vi "FUG_PowerSupply.SetCurrent.vi"(0 "i ref in":refnum<vi>, 2 "value":dbl, 5 "error in (no error)":errorcluster, 7 "channel":i32) -> (14 "i ref out":refnum<vi>, 19 "error out (no error)":errorcluster)   [LabVIEW 2014, in "FUG_PowerSupply.lvlib"]
doc: "This VI calculates the right current from the DB values, saves the actual set current to the I-Attribute and set´s the Set Current-Service."
uses:
  FUG_PowerSupply.lvlib
  CS_Core/CSSystem/CoreDefs/CoreDefs.error_type.ctl
  CS_Core/CSSystem/CoreDefs/CoreDefs.error_severity.ctl
  CS_Core/CSApplicationBaseClasses/PSChannelBase/PSChannelBase.directionType.ctl
  CS_Core/CSApplicationBaseClasses/PSChannelBase/PSChannelBase.serviceType.ctl
  CSlibraries/UtilityLib/UtilityLib.valueStatus.ctl
  CS_Core/CSSystem/CoreLib/CoreLib.lvlib
  CSlibraries/UtilityLib/UtilityLib.lvlib
  CS_Core/CSApplicationBaseClasses/PSChannelBase/PSChannelBase.lvlib
  CSlibraries-extern/DimLVEvent/LVDimInterface/LVDimInterface.lvlib
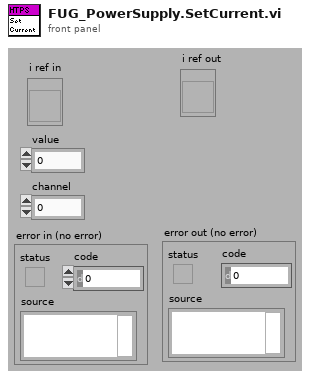
[diagram p1: front panel]
types:
  T1 = typedef "CoreDefs.error_severity.ctl" = enum16{"undefined", "information", "warning", "error", "fatal"}
  T2 = typedef "CoreDefs.error_type.ctl" = enum16{"no error", "can't load process", "can't unload process", "process does not exist", "can't install process", "can't remove process", "unknown function", "time out", "can't execute function", "duplicate queue name", "super not found", "caller queue invalid", "can't ping process", "unknown error", "VISA Error", "VISA timeout", "GPIB timeout", "GPIB error", "communication error", "data type mismatch", "can't read data from OPC server", "can't write data to OPC server", "OET error", "function not implemented", "process already exists", "invalid Shared Variable name", "error writing Shared Variable", "error reading Shared Variable", "invalid client name", "corrupt database", "unknown class", "call not authorized", "parameter out of range", "OET timeout: can't get data to modify", "invalid queue name", "requested operation incompatible with current state", "event undefined", "event disabled", "state undefined", "caller is not a friend", "EventBuilder: bad eventID", "EventBuilder: no DAQ devices", "a thread must not stop itself", "UNUSED ELEMENT4", "DiscArchiver: eventData incomplete", "DiscArchiver: eventData does not belong to run", "DiscArchiver: can't open file", "DiscArchiver: can't write to file", "DiscArchiver: available disc space low", "can't acquire semaphore", "error reading data from database", "notifier object is not existing", "can't register process", "can't unregister process", "illegal event type", "object disabled", "object already exists", "can't change state", "Instrument not found", "no connection to remote node", "invalid reference", "N/A", "UNUSED ELEMENT 1", "element not found", "illegal TCP/IP connection detected", "object does not exist", "invalid access ID", "unknown CS system", "invalid privilige", "unsupported data type", "unsupported server type", "IO server already exists", "Shared Variable already exists"}
  T3 = typedef "UtilityLib.lvlib/UtilityLib.valueStatus.ctl" = enum16{"no info available", "stand by/off", "on", "warning", "alarm/malfunction", "not implemented", "user action required", "important information", "system default", "control default", "indicator default", "button default"}
  T4 = typedef "PSChannelBase.lvlib/PSChannelBase.serviceType.ctl" = enum16{"onOff", "voltage", "current", "tripCurrent", "rampUpSpeed", "rampDownSpeed", "status"}
  T5 = typedef "PSChannelBase.lvlib/PSChannelBase.directionType.ctl" = enum16{"unknown", "update actual value", "update nominal value", "update both"}
  T6 = typedef "FUG_PowerSupply.lvlib/FUG_PowerSupply.i attribute.ctl" = cluster{"Type":string, "Elektrode Name":string, "CALC_FACTOR_SET_VOLTAGE":dbl, "CALC_FACTOR_GET_VOLTAGE":dbl, "CALC_FACTOR_GET_CURRENT":dbl, "CALC_FACTOR_SET_CURRENT ":dbl, "REG_VALUE":dbl, "Sign":bool, "setVoltID":i32, "setCurrentID":i32, "setPowerOnID":i32, "MaxVoltage":dbl}
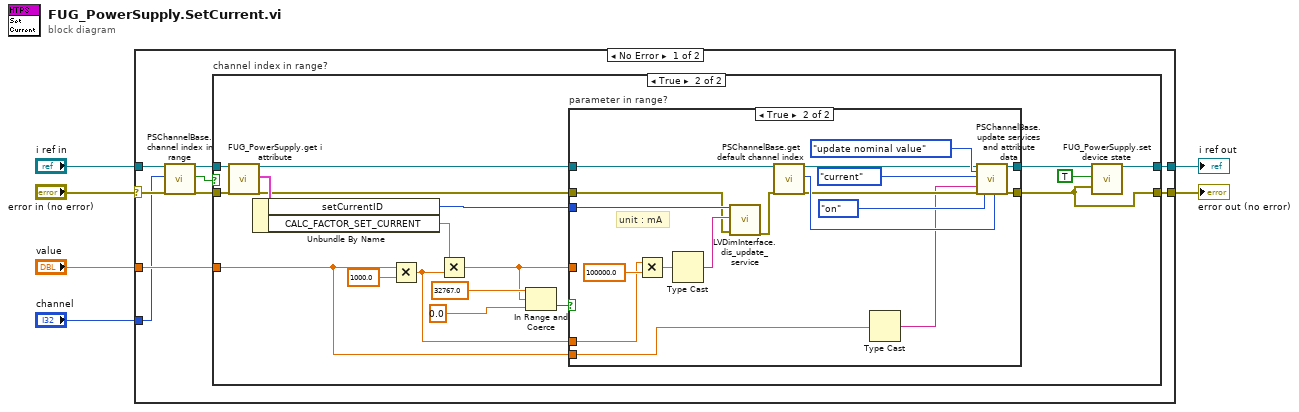
[diagram p0: block diagram]
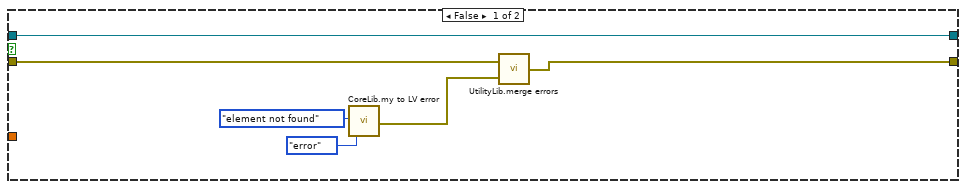
[diagram p2: hidden frame]
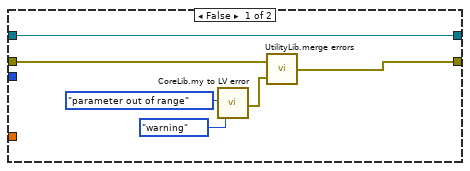
[diagram p3: hidden frame]
diagram:
  n1 = case shown="No Error" "error in (no error)" {
    selector: "error in (no error)" -> [w12 w65]
    tunnel: [w14 w65] -> w3
    tunnel: "i ref in" -> [w9 w64]
    tunnel: [w15 w64] -> w5
    tunnel: "value" -> [w13 _]
    tunnel: "channel" -> [w8 _]
    frame No Error {
      n2 = call "PSChannelBase.channel index in range.vi"("i ref in"=w9, "channelIndex"=w8, "error in (no error)"=w12) -> ("i ref out"=w10:refnum<vi>, "in range"=w7:bool, "error out"=w11:errorcluster)  [unwired: 14 in]
      n3 = case "channel index in range?" shown="True" w7 {
        tunnel: [w21 w26] -> w15
        tunnel: [w16 w25] -> w14
        tunnel: w13 -> [_ w22]
        tunnel: w11 -> [w18 w30]
        tunnel: w10 -> [w21 w29]
        frame False {
          n4 = call "CoreLib.my to LV error.vi"("ErrorTypes"=CoreDefs.error_type."element not found", "severityLevel"=CoreDefs.error_severity."error") -> ("myErrorCluster"=w17:errorcluster)  [unwired: 16 in, 1 out]
          n5 = call "UtilityLib.merge errors.vi"("error2 (no error)"=w17, "error1 (no error)"=w18) -> ("error out"=w16:errorcluster)
        }
        frame True {
          n6 = call "FUG_PowerSupply.get i attribute.vi"("i ref in"=w29, "error in (no error)"=w30) -> ("i ref out"=w33:refnum<vi>, "i attribute"=w39:T6, "error out"=w31:errorcluster)  [unwired: 15 in]
          n7 = Unbundle By Name(w39) -> ("setCurrentID"=w32:i32, "CALC_FACTOR_SET_CURRENT"=w34:dbl)
          n8 = Multiply(x=w22, y=1000.0) -> (x*y=w23:dbl)
          n9 = Multiply(x=w34, y=w23) -> (x*y=w35:dbl)
          n10 = In Range and Coerce(upper limit=32767.0, x=w35, lower limit=0.0 ("upper limit")) -> (In Range?=w38:bool)  [unwired: 1 out]
          n11 = case "parameter in range?" shown="True" w38 {
            tunnel: w31 -> [w42 w51]
            tunnel: [w40 w62] -> w25
            tunnel: w35 -> [_ _]
            tunnel: w33 -> [w45 w58]
            tunnel: [w45 w63] -> w27
            tunnel: w32 -> [_ w53]
            tunnel: w23 -> [_ w47]
            tunnel: w22 -> [_ w46]
            frame False {
              n12 = call "CoreLib.my to LV error.vi"("ErrorTypes"=CoreDefs.error_type."parameter out of range", "severityLevel"=CoreDefs.error_severity."warning") -> ("myErrorCluster"=w41:errorcluster)  [unwired: 16 in, 1 out]
              n13 = call "UtilityLib.merge errors.vi"("error2 (no error)"=w41, "error1 (no error)"=w42) -> ("error out"=w40:errorcluster)
            }
            frame True {
              # "unit : mA"
              n14 = Multiply(x=w47, y=100000.0) -> (x*y=w48:dbl)
              n15 = Type Cast(x=w48) -> (*(type *) &x=w52:string)  [unwired: 1 in]
              n16 = call "LVDimInterface.dis_update_service.vi"("my_serviceID"=w53, "data"=w52, "error in (no error)"=w51) -> ("error out"=w50:errorcluster)  [unwired: 14 in, 2 out]
              n17 = call "PSChannelBase.get default channel index.vi"("i ref in"=w58, "error in (no error)"=w50) -> ("i ref out"=w54:refnum<vi>, "defaultChannelIndex"=w57:i32, "error out"=w56:errorcluster)  [unwired: 15 in]
              n18 = Type Cast(x=w46) -> (*(type *) &x=w55:string)  [unwired: 1 in]
              n19 = call "PSChannelBase.update services and attribute data.vi"("i ref in"=w54, "direction"=PSChannelBase.directionType."update nominal value", "service"=PSChannelBase.serviceType."current", "value"=w55, "error in (no error)"=w56, "quality"=UtilityLib.valueStatus."on", "channelNumber"=w57) -> ("i ref out"=w63:refnum<vi>, "error out"=w62:errorcluster)  [unwired: 10 in, 1 out]
            }
          }
          n20 = call "FUG_PowerSupply.set device state.vi"("i ref in"=w27, "implicit"=TRUE, "device error"=w25) -> ("i ref out"=w26:refnum<vi>)  [unwired: 14 in, 2 out]
        }
      }
    }
    frame Error {
    }
  }
  "error out (no error)" <- w3
  "i ref out" <- w5
